vi "RemoveEdgePoint.vi"(2 "error constant":errorcluster, 3 "index":i32, 4 "array":cluster{"Edge Info":T1, "Boolean":bool}[](array[cluster]) {"Edge Info"."Distance (Real-World)" format="%.2f"; "Edge Info"."Location (Real-World)"."Y" format="%.2g"; "Edge Info"."Location (Real-World)"."X" format="%.2f"; "Edge Info"."Noise" format="%.2f"; "Edge Info"."Location (Pixel)"."Y" format="%.2g"; "Edge Info"."Location (Pixel)"."X" format="%.2f"; "Edge Info"."Strength" format="%.2f"; "Edge Info"."Distance (Pixel)" format="%.2f"}) -> (0 "error constant 2":errorcluster, 1 "output array":cluster{"Edge Info":T1, "Boolean":bool}[](array[cluster]) {"Edge Info"."Distance (Real-World)" format="%.2f"; "Edge Info"."Location (Real-World)"."Y" format="%.2g"; "Edge Info"."Location (Real-World)"."X" format="%.2f"; "Edge Info"."Noise" format="%.2f"; "Edge Info"."Location (Pixel)"."Y" format="%.2g"; "Edge Info"."Location (Pixel)"."X" format="%.2f"; "Edge Info"."Strength" format="%.2f"; "Edge Info"."Distance (Pixel)" format="%.2f"})   [LabVIEW 2015]
uses:
  <vilib>/vision/Measure.llb/Edge New.ctl
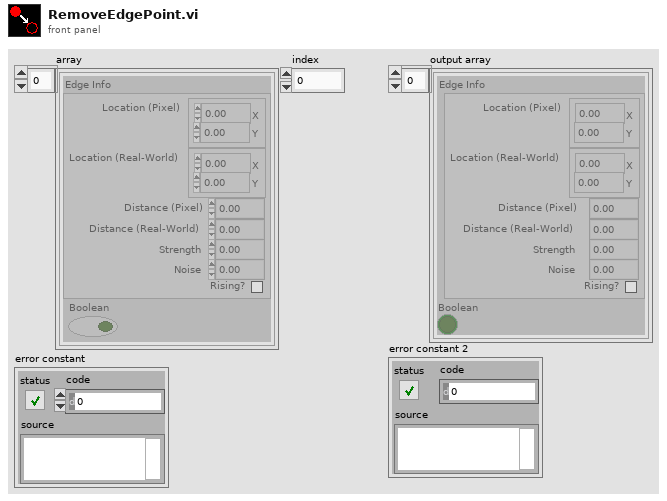
[diagram p1: front panel]
types:
  T1 = typedef "Edge New.ctl" = cluster{"Location (Pixel)":cluster{"X":sgl, "Y":sgl}, "Location (Real-World)":cluster{"X":sgl, "Y":sgl}, "Distance (Pixel)":dbl, "Distance (Real-World)":dbl, "Strength":dbl, "Noise":dbl, "Rising?":bool}
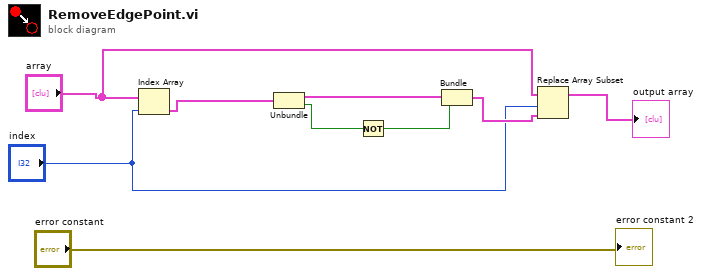
[diagram p0: block diagram]
diagram:
  n1 = Index Array(array="array", index="index") -> (element=w9:cluster{"Edge Info":T1, "Boolean":bool})
  n2 = Unbundle(w9) -> ("Edge Info"=w6:T1, "Boolean"=w8:bool)
  n3 = Not(x=w8) -> (.not. x?=w7:bool)
  n4 = Bundle("Edge Info"=w6, w7) -> (w5:cluster{"Edge Info":T1, bool})  [unwired: 1 in]
  n5 = Replace Array Subset(array="array", new element=w5, index="index") -> (→"output array":cluster{"Edge Info":T1, "Boolean":bool}[])
  "error constant 2" <- "error constant"
